vi "NTPModify2Origin.vi"() -> ()   [LabVIEW 2023]
uses:
  <vilib>/Utility/file.llb/Write Delimited Spreadsheet (I64).vi
panel:
  out "last Date":string
  out "tmp64bit":i64[](array[numeric])
  out "My std":dbl[](array[numeric]) format="%#_4g"
  out "Mean":dbl format="%.1f"
  out "Std":dbl format="%#_3g"
  out "Waveform Chart 4":dbl[][](graph) caption="Waveform Chart"
  out "Waveform Chart 3":dbl[][](graph) caption="Waveform Chart"
  out "Waveform Chart 2":i64[][](graph) caption="Waveform Chart"
  in  "Statistic":bool
  out "StDeviation":dbl[](array[numeric]) format="%#_4g"
  in  "Matches Tab":enum32{"Page 1", "Page 2"}(tab)
  out "Table Control":string[][](table)
  out "appended array":string[](array[string])
  out "Mean by row":dbl[](array[numeric]) format="%.2f"
  out "Variance (xi - x) by row of 6@49":dbl[][](array[numeric])
  out "Last Draw":i64[](array[numeric])
  out "Matches":i32[][](array[numeric])
  out "Matches":i32[](array[numeric])
  out "Last Suppose":i32[][](array[numeric])
  out "Indicator":bool
  in  "Deviation":bool
  in  "Check":bool
  in  "Play":bool
  out "Your Suppose":i32[][](array[numeric])
  out "Waveform Chart":i64[][](graph)
  in  "Stop":bool
  # "Last Draw"
  # "Last Suppose"
  # "Last Suppose"
  # "Suppose Graph"
  # "Std Deviation"
  # "6@49"
  # "Your Suppose"
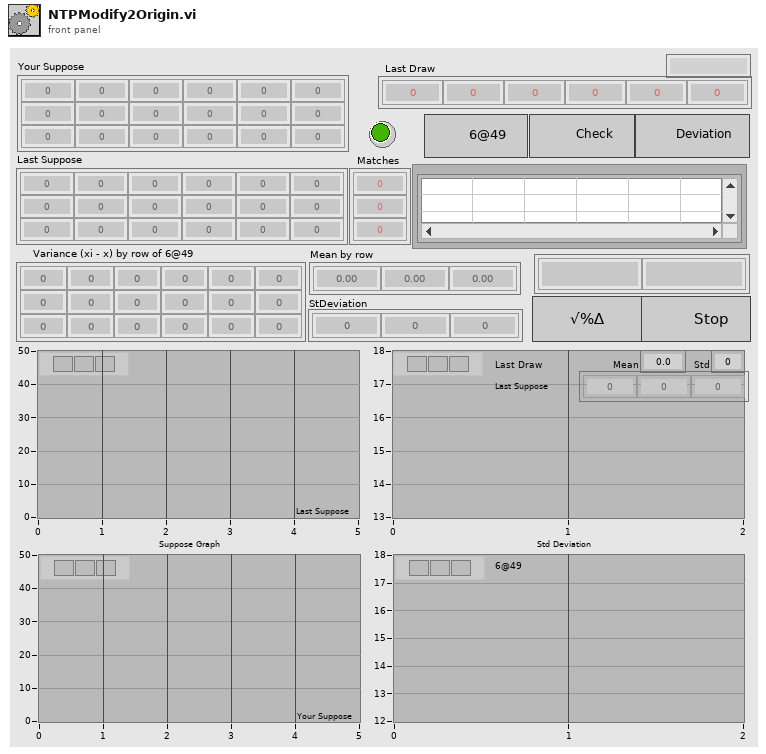
[diagram p1: front panel]
types:
  T1 = enum8{"Enabled", "Disabled", "Disabled and Grayed Out"}
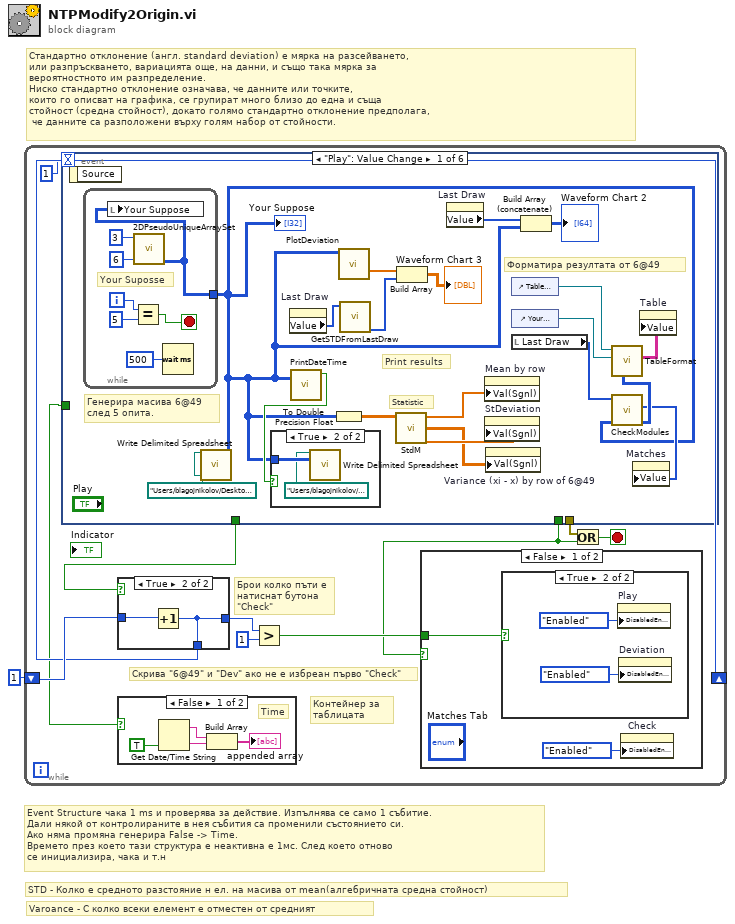
[diagram p0: block diagram]
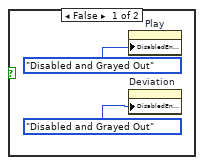
[diagram p4: hidden frame]
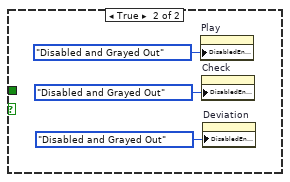
[diagram p5: hidden frame]
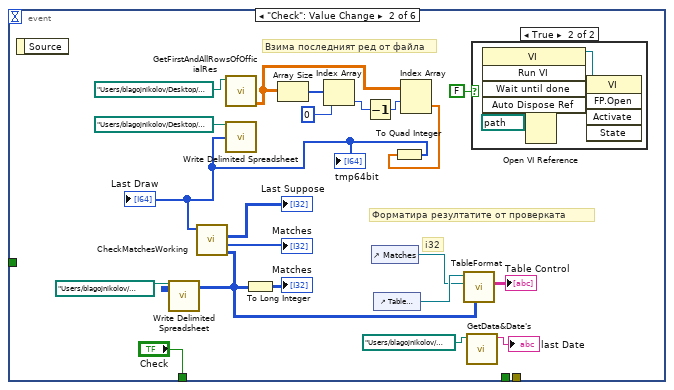
[diagram p7: hidden frame]
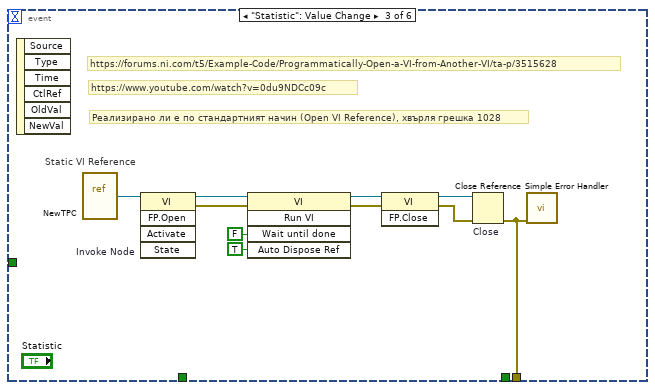
[diagram p9: hidden frame]
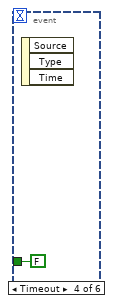
[diagram p10: hidden frame]
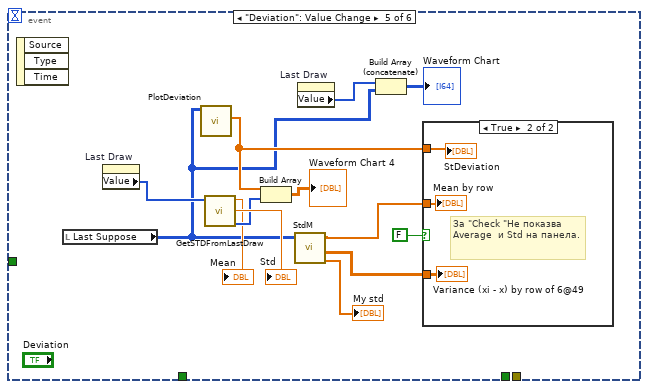
[diagram p11: hidden frame]
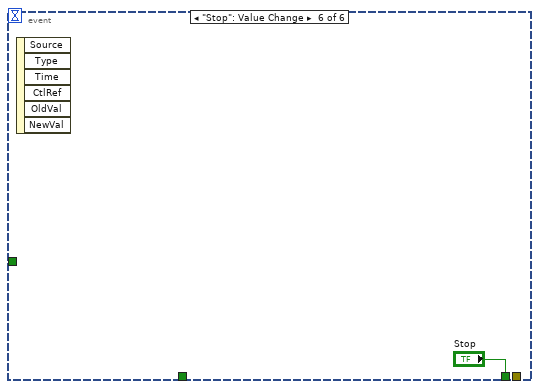
[diagram p13: hidden frame]
diagram:
  # "Varoance - С колко всеки елемент е отместен от средният"
  # "STD - Колко е средното разстояние н ел. на масива от mean(алгебричната средна стойност)"
  # "Event Structure чака 1 ms и проверява за действие. Изпълнява се само 1 събитие.\nДали някой от контролираните в нея събития са променили състоянието си.\nАко няма промяна генерира False -> Time.\nВремето през което тази структура е неактивна е 1мс. След което отново\nсе инициализира, чака и т.н"
  # "Стандартно отклонение (англ. standard deviation) е мярка на разсейването, \nили разпръскването, вариацията още, на данни, и също така мярка за \nвероятностното им разпределение. \nНиско стандартно отклонение означава, че данните или точките, \nкоито го описват на графика, се групират много близо до една и съща \nстойност (средна стойност), докато голямо стандартно отклонение предполага,\n че данните са разположени върху голям набор от стойности."
  n1 = while {
    shift-right: [w9] -> _
    shift-left: i64 1 -> [w11]
    stop <- w2 stop-if-true
    # "Скрива \"6@49\" и \"Dev\" ако не е избреан първо \"Check\""
    # "Брои колко пъти е\nнатиcнат бутона\n\"Check\""
    # "Контейнер за\nтаблицата"
    n2 = event shown="[0] \"Play\": Value Change" {
      selector: _ -> [_ _ _ _ _ _]
      dyn-events: _ -> [_ _ _ _ _ _]
      timeout: 1 -> [_ _ _ _ _ _]
      tunnel: [_ _ _ FALSE _ _] -> w6
      tunnel: [_ _ _ _ _ "Stop"] -> w4
      tunnel: [_ "Check" _ _ _ _] -> w5
      tunnel: [_ _ w83 _ _ _] -> w3
      event "Play": Value Change {
        # "Statistic"
        # "Форматира резултата от 6@49"
        # "Генерира масива 6@49\nслед 5 опита."
        # "Print results"
        n3 = event-data() -> ()  [unwired: 1 in, 1 out]
        n4 = while {
          tunnel: [w51] -> w29
          i -> [w55]
          stop <- w53 stop-if-true
          # "Your Suposse"
          n5 = Equal?(x=w55, y=5) -> (x = y?=w53:bool)
          n6 = call "2DPseudoUniqueArraySet.vi"("Colums"=6, "Rows"=3) -> ("2D Double Array"=w51:i32[][])  [unwired: 8 in, 1 out]
          n7 = local write "Your Suppose"(w51) -> ()
          n8 = Wait (ms)(milliseconds to wait=u32 500) -> ()  [unwired: 1 out]
        }
        "Your Suppose" <- w29
        n9 = call-poly <vilib>:"Write Delimited Spreadsheet.vi"("file path (dialog if empty)"=path "/Users/blagojnikolov/Desktop/@tmp/tmp649Gen.txt", "2D data"=w29) -> ()  [unwired: 12 in, 2 out]
        n10 = property on="Last Draw" class="Arr (strict)"() -> ("Value"=w40:i64[])  [unwired: 2 in, 2 out]
        n11 = call "PrintDateTime.vi"("2D"=w29) -> ("T button?"=w46:bool)  [unwired: 10 in]
        n12 = case shown="True" w46 {
          tunnel: w29 -> [_ w49]
          frame False {
          }
          frame True {
            n13 = call-poly <vilib>:"Write Delimited Spreadsheet.vi"("file path (dialog if empty)"=path "/Users/blagojnikolov/Desktop/@tmp/archive.txt", "2D data"=w49) -> ()  [unwired: 12 in, 2 out]
          }
        }
        n14 = To Double Precision Float(number=w29) -> (double precision float=w30:dbl[][])
        n15 = call "PlotDeviation.vi"("Array"=w29) -> ("STD"=w43:dbl[])  [unwired: 7 in, 3 out]
        n16 = call "GetSTDFromLastDraw.vi"("Officials Results"=w40) -> ("StdRes array"=w42:u64[])  [unwired: 8 in, 2 out]
        n17 = call "StdM.vi"("2D"=w30) -> ("My std"=w32:dbl[], "[Xi-X]"=w31:dbl[][], "Mean"=w33:dbl[])  [unwired: 6 in, 2 out]
        n18 = Build Array(w43, w42) -> (→"Waveform Chart 3":dbl[][])
        n19 = property on="Last Draw" class="Arr (strict)"() -> ("Value"=w44:i64[])  [unwired: 2 in, 2 out]
        n20 = property on="Mean by row" class="Arr (strict)"("Val(Sgnl)"=w33) -> ()  [unwired: 2 in, 2 out]
        n21 = property on="StDeviation" class="Arr (strict)"("Val(Sgnl)"=w32) -> ()  [unwired: 2 in, 2 out]
        n22 = property on="Variance (xi - x) by row of 6@49" class="Arr (strict)"("Val(Sgnl)"=w31) -> ()  [unwired: 2 in, 2 out]
        n23 = control-ref of="Table Control"() -> (w39:refnum<vi>)
        n24 = control-ref of="Your Suppose"() -> (w35:refnum<vi>)
        n25 = local read "Last Draw"() -> (w34:i64[])
        n26 = Build Array (concatenate)(w44, w29) -> (→"Waveform Chart 2":i64[][])
        n27 = call "CheckModules.vi"("Your Suppose"=w29, "Last Draw"=w34) -> ("Matches"=w37:i32[][], "Matches 2"=w36:i32[])  [unwired: 8 in]
        n28 = call "TableFormat.vi"("2D Double Array"=w37, "Arr Refnum"=w35, "Table in"=w39) -> ("TxtArray"=w38:string[][])  [unwired: 8 in]
        n29 = property on="Matches" class="Arr (strict)"("Value"=w36) -> ()  [unwired: 2 in, 2 out]
        n30 = property on="Table" class="Tbl (strict)"("Value"=w38) -> ()  [unwired: 2 in, 2 out]
      }
      event "Check": Value Change {
        # "Взима последният ред от файла"
        # "Форматира резултатите от проверката"
        # "i32"
        n31 = event-data() -> ()  [unwired: 1 in, 1 out]
        n32 = call "GetFirstAndAllRowsOfOfficialRes.vi"("file (use dialog)"=path "/Users/blagojnikolov/Desktop/@tmp/results.txt" ("file path (dialog if empty)")) -> ("All Officials Result"=w67:dbl[][])  [unwired: 8 in, 2 out]
        n33 = Array Size(array=w67) -> (size(s)=w65:i32[])
        n34 = Index Array(array=w65, index=0) -> (element=w66:i32)
        n35 = Decrement(x=w66) -> (x-1=w64:i32)
        n36 = control-ref of="Matches"() -> (w72:refnum<vi>)
        n37 = control-ref of="Table Control"() -> (w74:refnum<vi>)
        n38 = Index Array "Index Array"(array=w67, index (row)=w64) -> (element=w63:dbl[])  [unwired: 1 in]
        n39 = To Quad Integer(1:w63) -> (0:w62:i64[])
        "Last Draw" <- w62
        "tmp64bit" <- w62
        n40 = call "CheckMatchesWorking.vi"("Последен тираж"=w62) -> (0:w61:i64[][], "Съвпадения"=→"Matches":i32[], "Залози"=→"Last Suppose":i32[][])  [unwired: 7 in, 1 out]
        n41 = call-poly <vilib>:"Write Delimited Spreadsheet.vi"("file path (dialog if empty)"=path "/Users/blagojnikolov/Desktop/@tmp/matches.txt", "2D data"=w61) -> ()  [unwired: 12 in, 2 out]
        n42 = call-poly <vilib>:"Write Delimited Spreadsheet.vi"("file path (dialog if empty)"=path "/Users/blagojnikolov/Desktop/@tmp/officialResults.txt", "1D data"=w62) -> ()  [unwired: 12 in, 2 out]
        n43 = To Long Integer(number=w61) -> (32bit integer=→"Matches":i32[][])
        n44 = call "TableFormat.vi"("2D Double Array"=w61, "Arr Refnum"=w72, "Table in"=w74) -> ("TxtArray"=→"Table Control":string[][])  [unwired: 8 in]
        n45 = call "GetData&Date's.vi"("file (use dialog)"=path "/Users/blagojnikolov/Desktop/@tmp/fromSite.txt") -> ("LastDate"=→"last Date":string)  [unwired: 8 in, 2 out]
        n46 = case shown="True" FALSE {
          frame False {
          }
          frame True {
            n47 = Open VI Reference(vi path=path "/Users/blagojnikolov/Library/Mobile Documents/com~apple~CloudDocs/» LabView/LabView/Project'24/Projects/649/subVI Tools/CollorCellsInTableOnly.vi") -> (vi reference=w79:refnum<vi>)  [unwired: 5 in, 1 out]
            n48 = invoke on="Invoke Node" class="VI" method="Run VI"(reference=w79) -> (reference out=w78:refnum<vi>)  [unwired: 4 in, 4 out]
            n49 = invoke on="Invoke Node" class="VI" method="FP.Open"(reference=w78) -> ()  [unwired: 4 in, 5 out]
          }
        }
      }
      event "Statistic": Value Change {
        # "Static VI Reference"
        # "Реализирано ли е по стандартният начин (Open VI Reference), хвърля грешка 1028"
        # "https://www.youtube.com/watch?v=0du9NDCc09c"
        # "https://forums.ni.com/t5/Example-Code/Programmatically-Open-a-VI-from-Another-VI/ta-p/3515628"
        n50 = event-data() -> ()  [unwired: 1 in, 6 out]
        n51 = vi-ref "NewTPC.vi"() -> (w82:refnum<vi>)
        n52 = invoke on="Invoke Node" class="VI" method="FP.Open"(reference=w82) -> (reference out=w90:refnum<vi>, error out=w89:errorcluster)  [unwired: 4 in, 3 out]
        n53 = invoke class="VI" method="Run VI"(reference=w90, error in=w89, "Wait until done"=TRUE ("Wait Until Done"), "Auto Dispose Ref"=FALSE ("Auto Dispose Reference")) -> (reference out=w86:refnum<vi>, error out=w85:errorcluster)  [unwired: 1 in, 3 out]
        n54 = invoke class="VI" method="FP.Close"(reference=w86, error in=w85) -> (reference out=w81:refnum<vi>, error out=w84:errorcluster)  [unwired: 1 in, 1 out]
        n55 = Close Reference "Close"(reference=w81, error in (no error)=w84) -> (error out=w83:errorcluster)
        n56 = call <vilib>:"Simple Error Handler.vi"("error in (no error)"=w83) -> ()  [unwired: 4 in, 5 out]
      }
      event Timeout {
        n57 = event-data() -> ()  [unwired: 1 in, 3 out]
      }
      event "Deviation": Value Change {
        n58 = event-data() -> ()  [unwired: 1 in, 3 out]
        n59 = local read "Last Suppose"() -> (w95:i32[][])
        n60 = property on="Last Draw" class="Arr (strict)"() -> ("Value"=w102:i64[])  [unwired: 2 in, 2 out]
        n61 = call "PlotDeviation.vi"("Array"=w95) -> ("STD"=w98:dbl[])  [unwired: 7 in, 3 out]
        n62 = call "GetSTDFromLastDraw.vi"("Officials Results"=w102) -> ("StdRes array"=w99:u64[], "STD"=→"Std":dbl, "Mean"=→"Mean":dbl)  [unwired: 8 in]
        n63 = Build Array(w98, w99) -> (→"Waveform Chart 4":dbl[][])
        n64 = call "StdM.vi"("2D"=w95) -> ("My std"=→"My std":dbl[], "[Xi-X]"=w93:dbl[][], "Mean"=w94:dbl[])  [unwired: 6 in, 2 out]
        n65 = property on="Last Draw" class="Arr (strict)"() -> ("Value"=w103:i64[])  [unwired: 2 in, 2 out]
        n66 = Build Array (concatenate)(w103, w95) -> (→"Waveform Chart":i64[][])
        n67 = case shown="True" FALSE {
          tunnel: w93 -> [_ w107]
          tunnel: w98 -> [_ w106]
          tunnel: w94 -> [_ w105]
          frame False {
          }
          frame True {
            # "За \"Check \"Не показва Average  и Std на панела."
            "Variance (xi - x) by row of 6@49" <- w107
            "Mean by row" <- w105
            "StDeviation" <- w106
          }
        }
      }
      event "Stop": Value Change {
        n68 = event-data() -> ()  [unwired: 1 in, 6 out]
      }
    }
    n69 = case shown="True" w5 {
      tunnel: [w17 w18] -> w10
      tunnel: [w17 w18] -> w9
      tunnel: w11 -> [w17 w19]
      frame False {
      }
      frame True {
        n70 = Increment(x=w19) -> (x+1=w18:i64)
      }
    }
    n71 = case shown="False" w6 {
      frame False {
        # "Time"
        n72 = Get Date/Time String(want seconds? (F)=TRUE) -> (date string=w14:string, time string=w15:string)  [unwired: 2 in]
        n73 = Build Array(w14, w15) -> (→"appended array":string[])
      }
      frame True {
      }
    }
    n74 = Greater?(x=w10, y=i64 1) -> (0:w12:bool)
    n75 = case shown="False" w4 {
      tunnel: w12 -> [w20 _]
      frame False {
        n76 = case shown="True" w20 {
          frame False {
            n77 = property on="Play" class="Bool"("DisabledEnum"=T1."Disabled and Grayed Out" ("Disabled")) -> ()  [unwired: 2 in, 2 out]
            n78 = property on="Deviation" class="Bool"("DisabledEnum"=T1."Disabled and Grayed Out" ("Disabled")) -> ()  [unwired: 2 in, 2 out]
          }
          frame True {
            n79 = property on="Play" class="Bool"("DisabledEnum"=T1."Enabled" ("Disabled")) -> ()  [unwired: 2 in, 2 out]
            n80 = property on="Deviation" class="Bool"("DisabledEnum"=T1."Enabled" ("Disabled")) -> ()  [unwired: 2 in, 2 out]
          }
        }
        n81 = property on="Check" class="Bool"("DisabledEnum"=T1."Enabled" ("Disabled")) -> ()  [unwired: 2 in, 2 out]
      }
      frame True {
        n82 = property on="Play" class="Bool"("DisabledEnum"=T1."Disabled and Grayed Out" ("Disabled")) -> ()  [unwired: 2 in, 2 out]
        n83 = property on="Check" class="Bool"("DisabledEnum"=T1."Disabled and Grayed Out" ("Disabled")) -> ()  [unwired: 2 in, 2 out]
        n84 = property on="Deviation" class="Bool"("DisabledEnum"=T1."Disabled and Grayed Out" ("Disabled")) -> ()  [unwired: 2 in, 2 out]
      }
    }
    n85 = Or(x=w3, y=w4) -> (x .or. y?=w2:bool)
  }
